vi "Add reset.vi"(10 "x":u32, 11 "Input":u32[](array[numeric])) -> (2 "Output":u32[](array[numeric]))   [LabVIEW 2016]
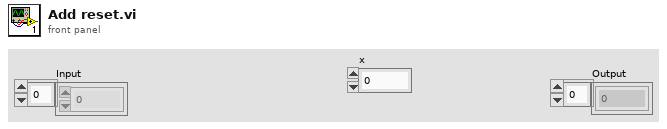
[diagram p1: front panel]
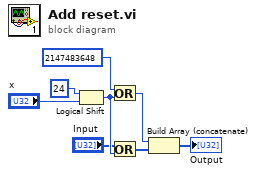
[diagram p0: block diagram]
diagram:
  n1 = Logical Shift(y=24, x="x") -> (x << y=w8:u32)
  n2 = Or(x=u32 2147483648 ("Color"), y=w8) -> (x .or. y?=w6:u32)
  n3 = Or(x="Input", y=w8) -> (x .or. y?=w5:u32[])
  n4 = Build Array (concatenate)(w6, w5) -> (→"Output":u32[])
